vi "createM1M3Settings.vi"(8 "error in (no error)":errorcluster, 11 "Boot in":refnum<class "Boot.lvclass">) -> (0 "error out":errorcluster, 2 "M1M3Settings":refnum<class "Setting.lvclass">, 3 "Boot out":refnum<class "Boot.lvclass">)   [LabVIEW 2016, in "Boot.lvclass"]
uses:
  Boot.lvclass
  Settings/Settings/Setting.lvclass
  Settings/M1M3SupportSettings/M1M3Settings.lvclass
  D:/Code/ts_M1M3Support/Settings/Settings/Setting.lvclass
  Settings/Settings/Setting.lvclass/Setting.ctl
  Boot.lvclass/Boot.ctl
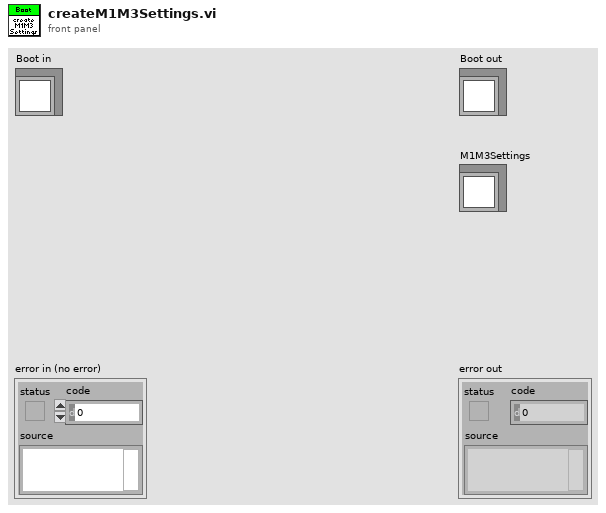
[diagram p1: front panel]
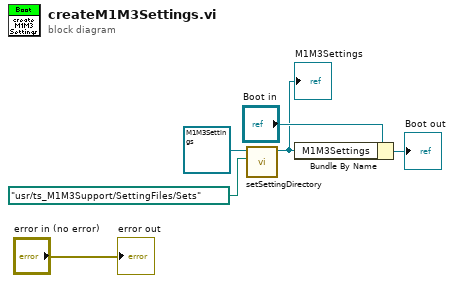
[diagram p0: block diagram]
diagram:
  n1 = call "setSettingDirectory.vi"("SettingDirectory"=path "/usr/ts_M1M3Support/SettingFiles/Sets", "BaseSetting in"=refnum<class "M1M3Settings.lvclass"> refnum ("M1M3Settings.lvclass")) -> ("BaseSetting out"=w2:refnum<class "M1M3Settings.lvclass">)  [unwired: 9 in]
  "M1M3Settings" <- w2
  n2 = Bundle By Name(cluster="Boot in", "M1M3Settings"=w2) -> (→"Boot out":refnum<class "Boot.lvclass">)
  "error out" <- "error in (no error)"
